vi "FPGA IP Chain V1.vi"() -> ()   [LabVIEW 2015]
uses:
  <vilib>/visionFPGA/Controls/IMAQ FPGA Image Size.ctl
  <vilib>/Platform/TimedLoop/XDataNode/timing_clust.ctl
  <vilib>/Platform/TimedLoop/XDataNode/nitl_modes.ctl
  <vilib>/Platform/TimedLoop/XDataNode/wakeup.ctl
  <vilib>/rvi/Emulation/niFpgaGetClockAttributes.vi
  <vilib>/rvi/Emulation/niFpgaSctlEmulationGetInTimedLoop.vi
  <vilib>/rvi/Emulation/niFpgaEmulationReportErrorSimple.vi
  <vilib>/rvi/Emulation/niFpgaCriticalErrorInLSC.vi
  <vilib>/visionFPGA/Basics/FIFO to Pixel Bus/IMAQ FPGA FIFO to Pixel Bus U8x1.vi
  <vilib>/visionFPGA/Basics/Pixel Bus to FIFO/IMAQ FPGA Pixel Bus to FIFO U1x1.vi
  <vilib>/rvi/Emulation/niFpgaEmulationIsFPGAContextNoSignature.vi
  <vilib>/rvi/errors/niFpgaSetErrorForExecOnDevCompSimple.vi
  <vilib>/rvi/eio/common/nirviEmuReportErrorAndStop.vi
  <vilib>/rvi/DataTransferAndStorage/Container/Common/niFpgaContainerGetUniqueNameForEmu.vi
  <vilib>/rvi/FIFO/Fifo_Resource/nirvififoEmulationSetSize.vi
  <vilib>/rvi/FIFO/Fifo_Resource/nirviFifoEmulationQueueMgr.vi
  <instcachedir>/0/nirviFifoEmulationQueueMgr_E5CAEC123FF24DC58D834DCA3CDAA9B5.lvgen/nirviFifoEmulationQueueMgr_E5CAEC123FF24DC58D834DCA3CDAA9B5_005.vi
  <vilib>/rvi/FIFO/Fifo_Resource/nirvififoEmulationDetermineInputValidOut.vi
  <vilib>/rvi/FIFO/Fifo_Resource/nirvififoEmulationCreateLock.vi
  <vilib>/rvi/Emulation/niFpgaProcessEmulError.vi
  <vilib>/rvi/FIFO/Fifo_Resource/nirvififoEmulationObtainLock.vi
  <vilib>/rvi/FIFO/Fifo_Resource/nirvififoEmulationReleaseLock.vi
  <vilib>/rvi/occurrence/nirviWaitOnOccurrenceBase.vi
  <vilib>/rvi/errors/nirviReportUnexpectedCaseInternalError.vi
  <vilib>/rvi/errors/nirviReportUnexpectedCaseInternalError (U32).vi
  <vilib>/rvi/interface/RandomDataEmulation/niFpgaRandomDataHandleErrors.vi
  <vilib>/rvi/Memory/Memory_Emulation/nirvimemoryFastEmulation.vi
  <vilib>/rvi/Memory/Memory_Emulation/nirvimemoryEmulation.vi
  <vilib>/Utility/error.llb/Clear Errors.vi
  <instcachedir>/0/nirviFifoEmulationQueueMgr_E5CAEC123FF24DC58D834DCA3CDAA9B5.lvgen/nirviFifoEmulationQueueMgr_E5CAEC123FF24DC58D834DCA3CDAA9B5_001.vi
  <instcachedir>/0/nirviFifoEmulationQueueMgr_E5CAEC123FF24DC58D834DCA3CDAA9B5.lvgen/nirviFifoEmulationQueueMgr_E5CAEC123FF24DC58D834DCA3CDAA9B5_003.vi
  <vilib>/Platform/TimedLoop/XDataNode/XDataNode.xnode
  <vilib>/rvi/DataTransferAndStorage/Container/XNode/niFpgaContainer.xnode
  <vilib>/rvi/FIFO/Fifo_Resource/nirvififoEmulationWrite.vi
  <vilib>/rvi/interface/RandomDataEmulation/nirviRandomDataFpgaReadWriteTemplate.vi
  <vilib>/rvi/FIFO/Fifo_Resource/nirvififoEmulationRead.vi
  <vilib>/rvi/FXPMathLib/FxpAdd/XNode/nifxpmath_Add.xnode
  <vilib>/Platform/TimedLoop/XDataNode/XDNodeRunTimeDep.lvlib
  <vilib>/visionFPGA/NI_VDM_FPGA_Basics.lvlib
  <vilib>/rvi/FXPMathLib/sim/FxpSim.dll
panel:
  out "Measured Pixels Counter":u32
  out "Yaccum":u32
  out "Xaccum":u32
  out "counter":u32
  out "ApCounter":u32
  in  "ResetAPCounter":bool
  in  "Range":cluster{"Lower Value":u8, "Upper Value":u8}={"Lower Value"=128, "Upper Value"=255}
  in  "Image Size":T1
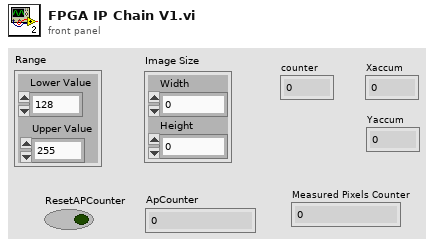
[diagram p1: front panel]
types:
  T1 = typedef "IMAQ FPGA Image Size.ctl" = cluster{"Width":u32, "Height":u32}
  T2 = typedef "XDNodeRunTimeDep.lvlib/timing_clust.ctl" = cluster{"Expected End [f-1]":u64, "Actual End [f-1]":u64, "Finished Late? [f-1]":bool, "Expected End [i-1]":u64, "Actual End [i-1]":u64, "Finished Late? [i-1]":bool, "Expected Start [i]":u64, "Actual Start [i]":u64, "Expected Start [f]":u64, "Actual Start [f]":u64, "Source Name":string, "Structure Name":string, "Period":i64, "Deadline":i64, "Offset":i64, "Start":i64, "Priority":i32, "Timeout":i32, "Mode":T3, "Wakeup Reason":T4, "Error":errorcluster, "Source Type":string, "Secondary Source Type":string, "Global End Time":u64, "Global Start Time":u64, "Frame Duration":u64, "Iteration Duration":u64, "Assigned CPU":i32, "I/O Scan Engine Mode":u32}
  T3 = typedef "XDNodeRunTimeDep.lvlib/nitl_modes.ctl" = enum32{"No Change", "Process missed periods, maintain original phase", "Discard missed periods, maintain original phase", "Process missed periods, ignore original phase", "Discard missed periods, ignore original phase"}
  T4 = typedef "XDNodeRunTimeDep.lvlib/wakeup.ctl" = enum32{"Normal", "Aborted", "Asynchronous wakeup", "Timing source error", "Timed loop error", "Timeout"}
  T5 = cluster{"Pixel Data":bool, "DV":bool, "EOL":bool, "EOI":bool, "Data Type":enum16{"U1 x 1"}}
  T6 = typedef "IMAQ FPGA Pixel Bus u8x1.ctl" = cluster{"Pixel Data":u8, "DV":bool, "EOL":bool, "EOI":bool, "Data Type":enum16{"U8 x 1"}}
  T7 = typedef "IMAQ FPGA Pixel Bus u1x1.ctl" = cluster{"Pixel Data":bool, "DV":bool, "EOL":bool, "EOI":bool, "Data Type":enum16{"U1 x 1"}}
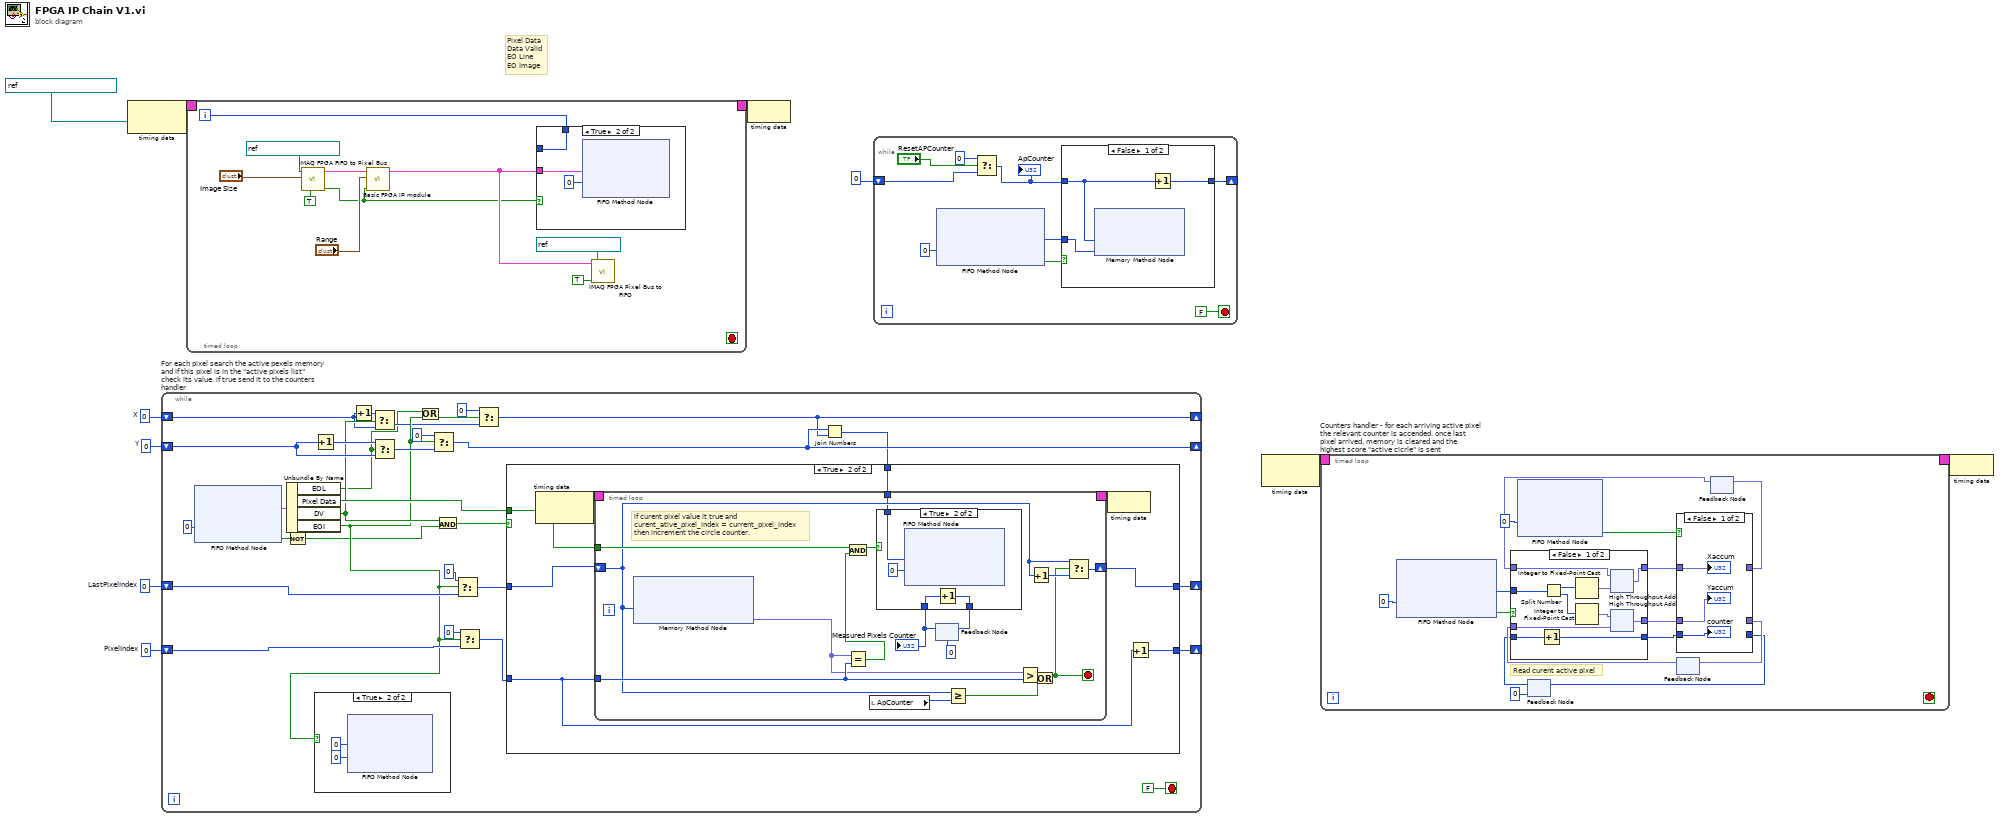
[diagram p0: block diagram]
diagram:
  w1 = u16 0  # X
  w2 = u16 0  # Y
  w6 = u32 0  # LastPixelIndex
  w7 = u32 0  # PixelIndex
  # "Pixel Data\nData Valid\nEO Line\nEO Image"
  n1 = node-c288(refnum<k21> "40 MHz Onboard Clock" ("Source Name")) -> (w10:T2)
  n2 = while "For each pixel search the active pexels memory and if this pixel is in the \"active pixels list\" check its value. if true send it to the counters handler" {
    shift-right: [w27] -> _
    shift-left: w7 -> [w28]
    shift-right: [w36] -> _
    shift-left: w6 -> [w37]
    shift-right: [w16] -> _
    shift-left: w2 -> [w26]
    shift-right: [w15] -> _
    shift-left: w1 -> [w21]
    stop <- FALSE stop-if-true
    n3 = xnode ("FIFO Method Node")("Timeout"=0) -> ("Element"=w32:T5, "Timed Out?"=w31:bool)  [unwired: 1 in, 1 out]
    n4 = Unbundle By Name(w32) -> ("EOL"=w12:bool, "Pixel Data"=w29:bool, "DV"=w22:bool, "EOI"=w19:bool)
    n5 = Not(x=w31) -> (.not. x?=w11:bool)
    n6 = Increment(x=w26) -> (x+1=w25:u16)
    n7 = case shown="True" w19 {
      frame False {
      }
      frame True {
        n8 = xnode ("FIFO Method Node")("Element"=u8 0, "Timeout"=0) -> ()  [unwired: 1 in, 2 out]
      }
    }
    n9 = Increment(x=w21) -> (x+1=w20:u16)
    n10 = Select(t=w20, s=w22, f=w21) -> (s? t:f=w18:u16)
    n11 = Select(t=w25, s=w12, f=w26) -> (s? t:f=w24:u16)
    n12 = Or(x=w12, y=w19) -> (x .or. y?=w13:bool)
    n13 = Select(t=u16 0, s=w19, f=w24) -> (s? t:f=w16:u16)
    n14 = And(x=w22, y=w11) -> (x .and. y?=w30:bool)
    n15 = Select(t=u32 0, s=w19, f=w37) -> (s? t:f=w35:u32)
    n16 = Select(t=u32 0, s=w19, f=w28) -> (s? t:f=w38:u32)
    n17 = Select(t=u16 0, s=w13, f=w18) -> (s? t:f=w15:u16)
    n18 = Join Numbers(hi=w16, lo=w15) -> ((hi.lo)=w14:u32)
    n19 = case shown="True" w30 {
      tunnel: w38 -> [w43 w52]
      tunnel: w35 -> [w44 w51]
      tunnel: [w44 w50] -> w36
      tunnel: w29 -> [_ w49]
      tunnel: [w43 w48] -> w27
      tunnel: w14 -> [_ w45]
      frame False {
      }
      frame True {
        n20 = node-c288() -> (w47:T2)  [unwired: 1 in]
        n21 = timed-loop {
          timing: w47 -> [_]
          timing-out: [_] -> w46
          tunnel: w52 -> [w64]
          shift-right: [w67] -> w50
          shift-left: w51 -> [w58]
          tunnel: w49 -> [w68]
          tunnel: w45 -> [w56]
          stop <- w61 stop-if-true
          # "if curent pixel value it true and \ncurent_ative_pixel_index = current_pixel_index\nthen increment the circle counter."
          n22 = xnode ("Memory Method Node")("Address"=w58) -> ("Data"=w57:fxp<+,19,19>)  [unwired: 1 in, 1 out]
          n23 = Equal?(x=w57, y=w64) -> (x = y?=w62:bool)
          n24 = And(x=w68, y=w62) -> (x .and. y?=w63:bool)
          n25 = local read "ApCounter"() -> (w60:u32)
          n26 = feedback #1(u32 0) -> (w55:u32)
          "Measured Pixels Counter" <- w55
          n27 = case shown="True" w63 {
            tunnel: w56 -> [_ w72]
            tunnel: w55 -> [w69 w71]
            tunnel: [w69 w70] -> w53
            frame False {
            }
            frame True {
              n28 = xnode ("FIFO Method Node")("Element"=w72, "Timeout"=0) -> ()  [unwired: 1 in, 2 out]
              n29 = Increment(x=w71) -> (x+1=w70:u32)
            }
          }
          n30 = feedback-in #1(w53) -> ()
          n31 = Greater Or Equal?(x=w58, y=w60) -> (x >= y?=w59:bool)
          n32 = Greater?(x=w57, y=w64) -> (0:w65:bool)
          n33 = Increment(x=w58) -> (x+1=w66:u32)
          n34 = Or(x=w65, y=w59) -> (x .or. y?=w61:bool)
          n35 = Select(t=w58, s=w61, f=w66) -> (s? t:f=w67:u32)
        }
        n36 = node-c288(w46) -> ()
        n37 = Increment(x=w52) -> (x+1=w48:u32)
      }
    }
  }
  n38 = timed-loop {
    timing: w10 -> [_]
    timing-out: [_] -> w9
    i -> [w78]
    stop <- _ stop-if-true
    n39 = call-poly <vilib>:"IMAQ FPGA FIFO to Pixel Bus.vi"("Ready For Output"=TRUE, "Image Size"="Image Size", "Source Image FIFO"=refnum<k21> "Source Image FIFO") -> ("Output Valid"=w81:bool, "Pixel Bus Out"=w85:T6)  [unwired: 6 in, 1 out]
    n40 = call "Basic FPGA IP module.vi"("Input Valid"=w81, "Range"="Range", "Red Plane Out"=w85) -> ("EdgeedPixels"=w82:T7)  [unwired: 4 in]
    n41 = case shown="True" w81 {
      tunnel: w82 -> [_ w89]
      tunnel: w78 -> [_ w88]
      tunnel: [_ w88] -> _
      frame False {
      }
      frame True {
        n42 = xnode ("FIFO Method Node")("Element"=w89, "Timeout"=0) -> ()  [unwired: 1 in, 2 out]
      }
    }
    n43 = call-poly <vilib>:"IMAQ FPGA Pixel Bus to FIFO.vi"("Input Valid"=TRUE, "Destination Image FIFO"=refnum<k21> "Dest Image FIFO", "Pixel Bus In"=w82) -> ()  [unwired: 8 in, 1 out]
  }
  n44 = node-c288(w9) -> ()
  n45 = while {
    shift-right: [w97] -> _
    shift-left: u32 0 -> [w95]
    stop <- FALSE stop-if-true
    n46 = xnode ("FIFO Method Node")("Timeout"=0) -> ("Element"=w98:u32, "Timed Out?"=w99:bool)  [unwired: 1 in, 1 out]
    n47 = Select(t=u32 0, s="ResetAPCounter", f=w95) -> (s? t:f=w94:u32)
    "ApCounter" <- w94
    n48 = case shown="False" w99 {
      tunnel: w98 -> [w102 _]
      tunnel: w94 -> [w103 w105]
      tunnel: [w104 w105] -> w97
      frame False {
        n49 = xnode ("Memory Method Node")("Address"=w103, "Data"=w102) -> ()  [unwired: 1 in, 1 out]
        n50 = Increment(x=w103) -> (x+1=w104:u32)
      }
      frame True {
      }
    }
  }
  n51 = node-c288() -> (w5:T2)  [unwired: 1 in]
  n52 = timed-loop "Counters handler - for each arriving active pixel the relevant counter is accended. once last pixel arrived, memory is cleared and the highest score \"active cicrle\" is sent" {
    timing: w5 -> [_]
    timing-out: [_] -> w4
    stop <- _ stop-if-true
    # "Read curent active pixel"
    n53 = xnode ("FIFO Method Node")("Timeout"=0) -> ("Element"=w117:u32, "Timed Out?"=w118:bool)  [unwired: 1 in, 1 out]
    n54 = xnode ("FIFO Method Node")("Timeout"=0) -> ("Timed Out?"=w114:bool)  [unwired: 1 in, 2 out]
    n55 = feedback #2(u16 0) -> (w109:u16)
    n56 = feedback #3() -> (w113:fxp<+,16,16>)  [unwired: 1 in]
    n57 = feedback #4() -> (w115:fxp<+,16,16>)  [unwired: 1 in]
    n58 = case shown="False" w118 {
      tunnel: w117 -> [w137 _]
      tunnel: [w136 w139] -> w116
      tunnel: w115 -> [w133 w139]
      tunnel: [w130 w140] -> w110
      tunnel: w113 -> [w129 w140]
      tunnel: w109 -> [w128 w138]
      tunnel: [w127 w138] -> w107
      frame False {
        n59 = Increment(x=w128) -> (x+1=w127:u16)
        n60 = Split Number(x=w137) -> (hi(x)=w135:u16, lo(x)=w132:u16)
        n61 = Integer to Fixed-Point Cast(integer=w135) -> (fixed-point=w134:fxp<+,16,16>)  [unwired: 1 in]
        n62 = Integer to Fixed-Point Cast(integer=w132) -> (fixed-point=w131:fxp<+,16,16>)  [unwired: 1 in]
        n63 = xnode ("High Throughput Add")("x"=w133, "y"=w134) -> ("x+y"=w136:fxp<+,16,16>)
        n64 = xnode ("High Throughput Add")("x"=w131, "y"=w129) -> ("x+y"=w130:fxp<+,16,16>)
      }
      frame True {
      }
    }
    n65 = case shown="False" w114 {
      tunnel: w116 -> [w123 w126]
      tunnel: [_ w126] -> w112
      tunnel: [_ w125] -> w111
      tunnel: w110 -> [w122 w125]
      tunnel: w107 -> [w121 w124]
      tunnel: [_ w124] -> w106
      frame False {
        "Xaccum" <- w123
        "Yaccum" <- w122
        "counter" <- w121
      }
      frame True {
      }
    }
    n66 = feedback-in #2(w106) -> ()
    n67 = feedback-in #3(w111) -> ()
    n68 = feedback-in #4(w112) -> ()
  }
  n69 = node-c288(w4) -> ()
